vi "LabVIEW FPGA FFT.vi"() -> ()   [LabVIEW 2020]
doc: "This FPGA VI illustrates use of the FFT in a single-cycle Timed Loop (SCTL). The FFT returns results in a \"burst\" fashion, requiring several calls on average for each valid output result.\n\nThe entire data pipeline uses a handshaking protocol to ensure that no data is lost, by throttling upstream nodes if any node is not ready to receive data. If the pipeline is too slow (as determined by the host VI DMA Read loop), the Sine Wave FIFO will eventually overflow, returning Timed Out? and notifies the host UI."
uses:
  <vilib>/Platform/TimedLoop/XDataNode/timing_clust.ctl
  <vilib>/Platform/TimedLoop/XDataNode/nitl_modes.ctl
  <vilib>/Platform/TimedLoop/XDataNode/wakeup.ctl
  <vilib>/rvi/Analysis/measure/FFT/simModelSupport/niFPGA FFT Sim Properties.ctl
  <vilib>/rvi/Analysis/measure/FFT/simModelSupport/niFPGA FFT Sim Types.ctl
  <vilib>/rvi/Analysis/measure/FFT/simModelSupport/niFpgaFFTSimArithmeticProperties.ctl
  <vilib>/rvi/Analysis/measure/FFT/simModelSupport/niFpgaFFTSimDfxp.ctl
  <vilib>/fxp/LVFixedPointQuantizationPolicyTypeDef.ctl
  <vilib>/rvi/DataTransferAndStorage/Container/Common/niFpgaContainerGetUniqueNameForEmu.vi
  <vilib>/rvi/DataTransferAndStorage/Container/Common/niFpgaContainerSetEmuInfo.vi
  <vilib>/rvi/eio/common/nirviEmuReportErrorAndStop.vi
  <vilib>/rvi/eio/common/nirviEmuTemplateMethod_errors.vi
  <vilib>/rvi/Emulation/niFpgaGetClockAttributes.vi
  <vilib>/rvi/Emulation/niFpgaSctlEmulationGetInTimedLoop.vi
  <vilib>/rvi/Emulation/niFpgaEmulationReportErrorSimple.vi
  <vilib>/rvi/DataTransferAndStorage/Container/Common/niFpgaContainerExecOnDevCompGetState.vi
  <vilib>/rvi/Emulation/niFpgaEmulationIsFPGAContextNoSignature.vi
  <vilib>/rvi/errors/niFpgaSetErrorForExecOnDevCompSimple.vi
  <vilib>/rvi/FIFO/Fifo_Resource/nirvififoEmulationSetSize.vi
  <vilib>/rvi/FIFO/Fifo_Resource/nirviFifoEmulationQueueMgr.vi
  <instcachedir>/0/nirviFifoEmulationQueueMgr_E5CAEC123FF24DC58D834DCA3CDAA9B5.lvgen/nirviFifoEmulationQueueMgr_E5CAEC123FF24DC58D834DCA3CDAA9B5_003.vi
  <vilib>/rvi/FIFO/Fifo_Resource/nirvififoEmulationDetermineInputValidOut.vi
  <vilib>/rvi/FIFO/Fifo_Resource/nirvififoEmulationCreateLock.vi
  <vilib>/rvi/Emulation/niFpgaProcessEmulError.vi
  <vilib>/rvi/FIFO/Fifo_Resource/nirvififoEmulationObtainLock.vi
  <vilib>/rvi/FIFO/Fifo_Resource/nirvififoEmulationReleaseLock.vi
  <vilib>/rvi/occurrence/nirviWaitOnOccurrenceBase.vi
  <vilib>/rvi/errors/nirviReportUnexpectedCaseInternalError.vi
  <vilib>/rvi/errors/nirviReportUnexpectedCaseInternalError (U32).vi
  <vilib>/Utility/error.llb/Clear Errors.vi
  <vilib>/rvi/interface/RandomDataEmulation/niFpgaRandomDataHandleErrors.vi
  <vilib>/rvi/Emulation/niFpgaCriticalErrorInLSC.vi
  <vilib>/rvi/Analysis/measure/FFT/simModelSupport/niFpgaFFTSimModelCore.vi
  <vilib>/Platform/TimedLoop/XDataNode/XDataNode.xnode
  <vilib>/rvi/LocalResourceManager/LocalResourceManager.xnode
  <vilib>/eio/EIONode/EIONode.xnode
  <vilib>/rvi/DataTransferAndStorage/Container/XNode/niFpgaContainer.xnode
  <vilib>/rvi/FIFO/Fifo_Resource/niFpgaFifoEmulationRefIn.vi
  <vilib>/rvi/interface/RandomDataEmulation/nirviRandomDataFpgaReadWriteTemplate.vi
  <vilib>/rvi/Analysis/measure/FFT/XNode/niFpgaFFT.xnode
  <vilib>/Platform/TimedLoop/XDataNode/XDNodeRunTimeDep.lvlib
panel:
  out "Overflow":bool
  out "Actual Sample Period (ticks)":u32
  out "Invalid Period":bool
  in  "Requested Sample Period (ticks)":u32=1000
  # "Overview: Demonstrates the use of the LabVIEW FPGA FFT function for custom in-hardware signal processing\nRequirements: LabVIEW FPGA Module, NI-RIO\nInstructions: Run the VI"
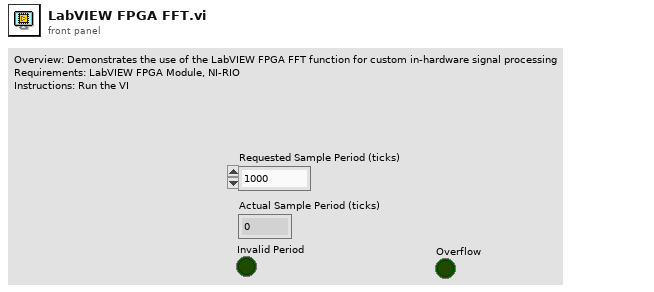
[diagram p1: front panel]
types:
  T1 = typedef "XDNodeRunTimeDep.lvlib/timing_clust.ctl" = cluster{"Expected End [f-1]":u64, "Actual End [f-1]":u64, "Finished Late? [f-1]":bool, "Expected End [i-1]":u64, "Actual End [i-1]":u64, "Finished Late? [i-1]":bool, "Expected Start [i]":u64, "Actual Start [i]":u64, "Expected Start [f]":u64, "Actual Start [f]":u64, "Source Name":string, "Structure Name":string, "Period":i64, "Deadline":i64, "Offset":i64, "Start":i64, "Priority":i32, "Timeout":i32, "Mode":T2, "Wakeup Reason":T3, "Error":errorcluster, "Source Type":string, "Secondary Source Type":string, "Global End Time":u64, "Global Start Time":u64, "Frame Duration":u64, "Iteration Duration":u64, "Assigned CPU":i32, "I/O Scan Engine Mode":u32}
  T2 = typedef "XDNodeRunTimeDep.lvlib/nitl_modes.ctl" = enum32{"No Change", "Process missed periods, maintain original phase", "Discard missed periods, maintain original phase", "Process missed periods, ignore original phase", "Discard missed periods, ignore original phase"}
  T3 = typedef "XDNodeRunTimeDep.lvlib/wakeup.ctl" = enum32{"Normal", "Aborted", "Asynchronous wakeup", "Timing source error", "Timed loop error", "Timeout"}
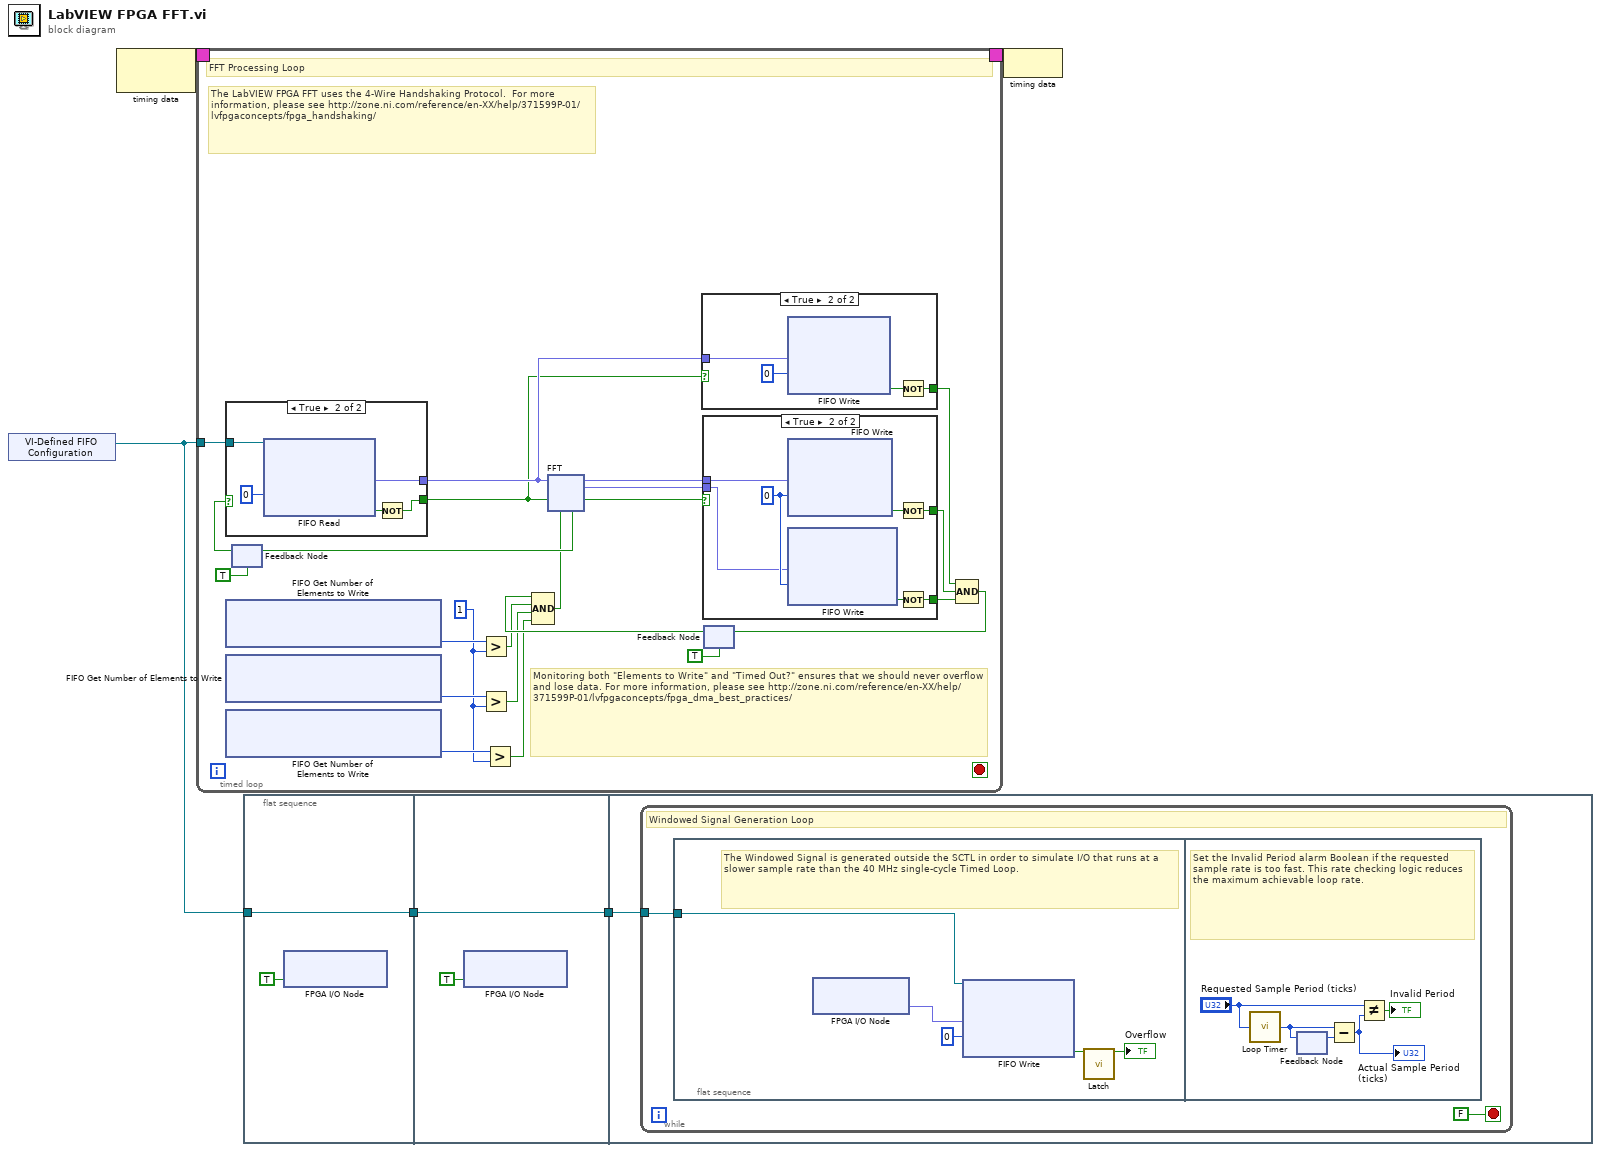
[diagram p0: block diagram]
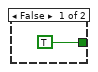
[diagram p2: hidden frame]
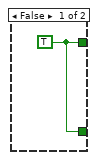
[diagram p3: hidden frame]
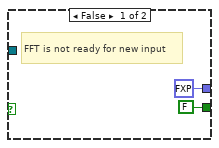
[diagram p4: hidden frame]
diagram:
  n1 = xnode "VI-Defined FIFO Configuration"() -> ("FIFO Out"=w3:refnum<k21>)
  n2 = node-c288() -> (w5:T1)  [unwired: 1 in]
  n3 = timed-loop {
    timing: w5 -> [_]
    timing-out: [_] -> w4
    tunnel: w3 -> [w24]
    stop <- _ stop-if-true
    w12 = u32 1 ("y")
    # "Monitoring both \"Elements to Write\" and \"Timed Out?\" ensures that we should never overflow and lose data. For more information, please see http://zone.ni.com/reference/en-XX/help/371599P-01/lvfpgaconcepts/fpga_dma_best_practices/"
    # "The LabVIEW FPGA FFT uses the 4-Wire Handshaking Protocol.  For more information, please see http://zone.ni.com/reference/en-XX/help/371599P-01/lvfpgaconcepts/fpga_handshaking/"
    # "FFT Processing Loop"
    n4 = xnode ("FIFO Get Number of Elements to Write")() -> ("Number of Elements to Write"=w15:u32)  [unwired: 1 in, 1 out]
    n5 = xnode ("FIFO Get Number of Elements to Write")() -> ("Number of Elements to Write"=w14:u32)  [unwired: 1 in, 1 out]
    n6 = xnode ("FIFO Get Number of Elements to Write")() -> ("Number of Elements to Write"=w13:u32)  [unwired: 1 in, 1 out]
    n7 = feedback #1(TRUE ("ready for input")) -> (w28:bool)
    n8 = case shown="True" w28 {
      tunnel: [FALSE w73] -> w25
      tunnel: [fxp<+/-,16,5> 0.0 ("Element") w74] -> w27
      tunnel: w24 -> [_ w70]
      frame False {
        # "FFT is not ready for new input"
      }
      frame True {
        n9 = xnode ("FIFO Read")("Timeout"=0, "FIFO In"=w70) -> ("Element"=w74:fxp<+/-,24,7>, "Timed Out?"=w72:bool)  [unwired: 1 out]
        n10 = Not(x=w72) -> (.not. x?=w73:bool)
      }
    }
    n11 = Greater?(x=w15, y=w12) -> (0:w9:bool)
    n12 = Greater?(x=w14, y=w12) -> (0:w8:bool)
    n13 = Greater?(x=w13, y=w12) -> (0:w7:bool)
    n14 = case shown="True" w25 {
      tunnel: w27 -> [_ w56]
      tunnel: [TRUE ("Timed Out?") w57] -> w20
      frame False {
      }
      frame True {
        n15 = xnode ("FIFO Write")("Element"=w56, "Timeout"=0) -> ("Timed Out?"=w58:bool)  [unwired: 1 in, 1 out]
        n16 = Not(x=w58) -> (.not. x?=w57:bool)
      }
    }
    n17 = feedback #2(TRUE) -> (w10:bool)
    n18 = Compound Arithmetic op=AND(w10, w9, w8, w7) -> (w11:bool)
    n19 = xnode "FFT"("real data in"=w27, "input valid"=w25, "ready for output"=w11) -> ("ready for input"=w26:bool, "real data out"=w23:fxp<+/-,32,16>, "imaginary data out"=w22:fxp<+/-,32,16>, "output valid"=w21:bool)  [unwired: 2 in, 1 out]
    n20 = feedback-in #1(w26) -> ()
    n21 = case shown="True" w21 {
      tunnel: w23 -> [_ w62]
      tunnel: w22 -> [_ w61]
      tunnel: [w60 w64] -> w19
      tunnel: [w60 w63] -> w18
      frame False {
        w60 = TRUE ("Timed Out?")
      }
      frame True {
        w67 = 0 ("Timeout")
        n22 = xnode ("FIFO Write")("Element"=w62, "Timeout"=w67) -> ("Timed Out?"=w66:bool)  [unwired: 1 in, 1 out]
        n23 = xnode ("FIFO Write")("Element"=w61, "Timeout"=w67) -> ("Timed Out?"=w65:bool)  [unwired: 1 in, 1 out]
        n24 = Not(x=w66) -> (.not. x?=w64:bool)
        n25 = Not(x=w65) -> (.not. x?=w63:bool)
      }
    }
    n26 = Compound Arithmetic op=AND(w20, w19, w18) -> (w17:bool)
    n27 = feedback-in #2(w17) -> ()
  }
  n28 = flat-sequence {
    tunnel: w3 -> [w78]
    tunnel: [w78] -> w1
    tunnel: [w80] -> w2
    tunnel: w1 -> [w80]
    tunnel: w2 -> [w81]
    frame #0 {
      n29 = xnode "FPGA I/O Node"("Mod1/Stop"=TRUE) -> ()  [unwired: 1 in, 1 out]
    }
    frame #1 {
      n30 = xnode "FPGA I/O Node"("Mod1/Start"=TRUE) -> ()  [unwired: 1 in, 1 out]
    }
    frame #2 {
      n31 = while {
        tunnel: w81 -> [w83]
        stop <- FALSE stop-if-true
        # "Windowed Signal Generation Loop"
        n32 = flat-sequence {
          tunnel: w83 -> [w86]
          frame #0 {
            # "The Windowed Signal is generated outside the SCTL in order to simulate I/O that runs at a slower sample rate than the 40 MHz single-cycle Timed Loop."
            n33 = xnode "FPGA I/O Node"() -> ("Mod1/AI0"=w84:fxp<+/-,24,7>)  [unwired: 1 in, 1 out]
            n34 = xnode ("FIFO Write")("Element"=w84, "Timeout"=0, "FIFO In"=w86) -> ("Timed Out?"=w85:bool)  [unwired: 1 out]
            n35 = call "Latch.vi"("Input"=w85) -> ("Output"=→"Overflow":bool)  [unwired: 14 in]
          }
          frame #1 {
            # "Set the Invalid Period alarm Boolean if the requested sample rate is too fast. This rate checking logic reduces the maximum achievable loop rate."
            n36 = call "Loop Timer"("Count(Ticks)"="Requested Sample Period (ticks)") -> ("Tick Count(Ticks)"=w89:u32)
            n37 = feedback #3() -> (w90:u32)  [unwired: 1 in]
            n38 = feedback-in #3(w89) -> ()
            n39 = Subtract(x=w89, y=w90) -> (x-y=w93:u32)
            "Actual Sample Period (ticks)" <- w93
            n40 = Not Equal?(x="Requested Sample Period (ticks)", y=w93) -> (x != y?=→"Invalid Period":bool)
          }
        }
      }
    }
  }
  n41 = node-c288(w4) -> ()
